vi "332 set setpoint.vi"(0 "Set Temperature SetPoint:332":dbl format="%.3f") -> ()   [LabVIEW 2012]
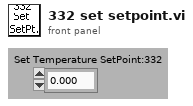
[diagram p1: front panel]
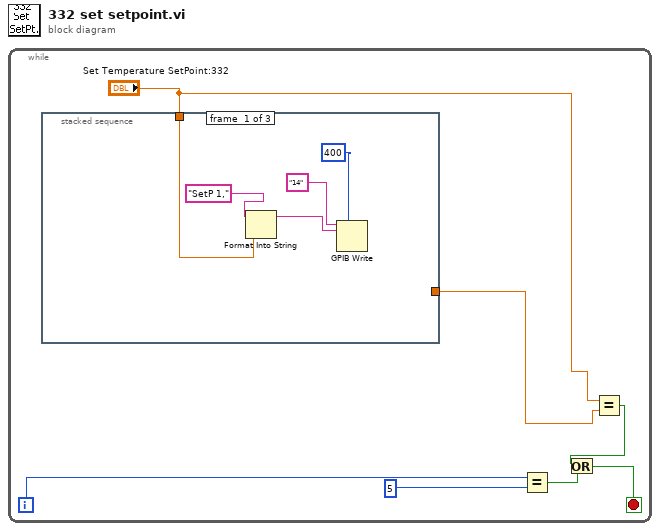
[diagram p0: block diagram]
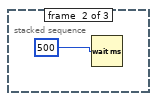
[diagram p2: hidden frame]
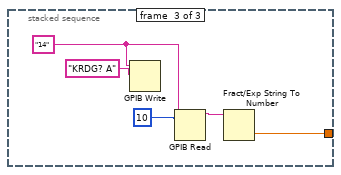
[diagram p3: hidden frame]
diagram:
  n1 = while {
    i -> [w1]
    stop <- w4 stop-if-true
    n2 = stacked-sequence {
      tunnel: "Set Temperature SetPoint:332" -> [w9 _ _]
      tunnel: [_ _ w14] -> w6
      frame #0 {
        n3 = Format Into String(initial string="SetP 1,", w9) -> (resulting string=w12:string)  [unwired: 2 in, 1 out]
        n4 = GPIB Write(0:"14", 1:w12, 4:400) -> ()  [unwired: 2 in, 2 out]
      }
      frame #1 {
        n5 = Wait (ms)(milliseconds to wait=500) -> ()  [unwired: 1 out]
      }
      frame #2 {
        w16 = "14"
        n6 = GPIB Write(0:w16, 1:"KRDG? A") -> ()  [unwired: 3 in, 2 out]
        n7 = GPIB Read(0:w16, 1:10) -> (5:w18:string)  [unwired: 3 in, 2 out]
        n8 = Fract/Exp String To Number(string=w18) -> (number=w14:dbl)  [unwired: 3 in, 1 out]
      }
    }
    n9 = Equal?(x=w1, y=5) -> (x = y?=w3:bool)
    n10 = Equal?(x="Set Temperature SetPoint:332", y=w6) -> (x = y?=w5:bool)
    n11 = Or(x=w5, y=w3) -> (x .or. y?=w4:bool)
  }
